vi "Display Mode Value.vi"(10 "Display Mode":T1) -> (2 "DisplayMode":u8 format="%.0x")   [LabVIEW 2023, in "CTI-Visa-DeviceLib.lvlib" / "LCD-I2C.lvclass"]
uses:
  LCD-I2C.lvclass
  Display Mode.ctl
  Entry Shift.ctl
  Glyph Entry.ctl
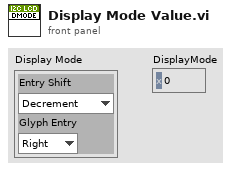
[diagram p1: front panel]
types:
  T1 = typedef "CTI-Visa-DeviceLib.lvlib/LCD-I2C.lvclass/Display Mode.ctl" = cluster{"Entry Shift":T2, "Glyph Entry":T3}
  T2 = typedef "CTI-Visa-DeviceLib.lvlib/LCD-I2C.lvclass/Entry Shift.ctl" = enum8{"Decrement", "Increment"}
  T3 = typedef "CTI-Visa-DeviceLib.lvlib/LCD-I2C.lvclass/Glyph Entry.ctl" = enum8{"Right", "Left"}
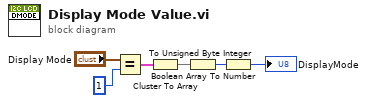
[diagram p0: block diagram]
diagram:
  n1 = Equal?(x="Display Mode", y=1) -> (x = y?=w4:cluster{"Entry Shift":bool, "Glyph Entry":bool})
  n2 = Cluster To Array(cluster=w4) -> (array=w3:bool[])
  n3 = Boolean Array To Number(Boolean array=w3) -> (number=w2:u32)
  n4 = To Unsigned Byte Integer(number=w2) -> (unsigned 8bit integer=→"DisplayMode":u8)
